vi "Autonomous Independent.vi"   [LabVIEW 2017]
doc: "This VI is called when autonomous begins, and will automatically be terminated when autonomous ends. You can carry out timed or sensor driven robot movement independently without needing to return to the caller."
uses:
  <vilib>/Rock Robotics/WPI/Utilities/WPI_GetSetVariantRefNum.vi
  <vilib>/Rock Robotics/Network Tables/NT Write Numeric Array.vi
  Robot Global Data.vi
  <vilib>/addons/control/pid/pid.llb/PID (DBL).vi
  <vilib>/addons/control/pid/NI_PID_pid.lvlib
panel:
  # "Be sure to right-click and choose Data Operations>>Make Current Value default if you want to save the array values with the VI"
types:
  T1 = typedef "WPI_JoystickDevRef.ctl" = cluster{"Device":T2}
  T2 = typedef "WPI_JoystickDeviceEnum.ctl" = enum16{"USB 0", "USB 1", "USB 2", "USB 3", "USB 4", "USB 5"}
  T3 = typedef "WPI_MotorControlDeviceRef.ctl" = cluster{"DeviceStatus":errorcluster, "Type":T4, "PWM":cluster{"PWM Channel":T5, "DeadBand":T6}, "CAN":cluster{"Device Number":u8, "SetOutput VI Ref":variant, "GetOutput VI Ref":variant, "Enable VI Ref":variant, "Disable VI Ref":variant, "Data":variant}, "Invert":bool, "DIO PWM":cluster{"PWM \"Enable\" Channel":T5, "DIOChannel":T7, "PWM Rate":dbl}}
  T4 = typedef "WPI_MotorControlType.ctl" = enum16{"PWM", "CAN", "DIO PWM"}
  T5 = typedef "FPGA_DIOPWMChannel.ctl" = enum8{"PWM 0", "PWM 1", "PWM 2", "PWM 3", "PWM 4", "PWM 5", "PWM 6", "PWM 7", "PWM 8", "PWM 9", "PWM MXP 0", "PWM MXP 1", "PWM MXP 2", "PWM MXP 3", "PWM MXP 4", "PWM MXP 5", "PWM MXP 6", "PWM MXP 7", "PWM MXP 8", "PWM MXP 9", "Invalid"}
  T6 = typedef "WPI_PWMDeadband.ctl" = cluster{"Name":string, "maxPositivePwm":i32, "minPositivePwm":i32, "centerPwm":i32, "maxNegativePwm":i32, "minNegativePwm":i32, "angularRange":u16}
  T7 = typedef "FPGA_DIOChannel.ctl" = enum8{"DIO 0", "DIO 1", "DIO 2", "DIO 3", "DIO 4", "DIO 5", "DIO 6", "DIO 7", "DIO 8", "DIO 9", "DIO MXP 0", "DIO MXP 1", "DIO MXP 2", "DIO MXP 3", "DIO MXP 4", "DIO MXP 5", "DIO MXP 6", "DIO MXP 7", "DIO MXP 8", "DIO MXP 9", "DIO MXP 10", "DIO MXP 11", "DIO MXP 12", "DIO MXP 13", "DIO MXP 14", "DIO MXP 15", "SPI Port CS1", "SPI Port CS2", "SPI Port CS3", "SPI Port MISO", "SPI Port MOSI", "Invalid"}
  T8 = cluster{"proportional gain (Kc)":dbl, "integral time (Ti, min)":dbl, "derivative time (Td, min)":dbl}
  T9 = typedef "CTRE_PigeonIMU_DeviceRef.ctl" = cluster{"DeviceStatus":errorcluster, "Device Number":u8, "Type":T10, "Device ID":u32, "Handle":u64, "UsageFrame":u32, "Library Path":path}
  T10 = typedef "CTRE_PigeonIMU_ConnectionType.ctl" = u32
  T11 = typedef "WPI_RobotDriveDevRef.ctl" = cluster{"DevStatus":errorcluster, "Motors[]":T3[], "Square Inputs":bool, "Max Output":dbl}
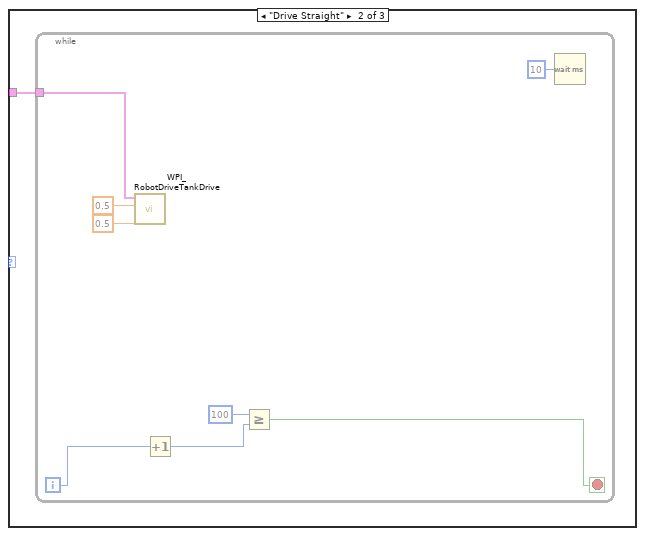
[diagram p2: hidden frame]
diagram:
  (unwired) "This function is run in parallel when the autonomous period begins. It will be terminated automatically when the period ends.\n\nNote that all Driver Station inputs are automatically latched and will not change once auto begins."
  # "This gives you the joystick value\nthat is often the throttle"
  # "Use time and/or sensors to control how the robot drives."
  n1 = call <vilib>:"WPI_JoystickRefNum Registry Get.vi"("refnum name"="Joystick 0") -> ("JoystickDevRef"=w21:T1)  [unwired: 1 in, 9 out]
  n2 = call <vilib>:"WPI_JoystickGetValues.vi"("JoystickDevRef"=w21) -> ("Buttons"=w19:bool[], "Axes"=w20:dbl[])  [unwired: 6 in, 3 out]
  n3 = call-poly <vilib>:"NT Write Value.vi"("Numeric Array"=w20, "Name"="Joystick 0/Axes") -> ()  [unwired: 9 in, 1 out]
  n4 = call <vilib>:"WPI_MotorControlRefNum Registry Get.vi"("refnum name"="LeftMaster") -> ("error out"=w14:errorcluster, "MotorControlDevRef"=w13:T3)  [unwired: 9 in]
  n5 = call <vilib>:"WPI_MotorControlRefNum Registry Get.vi"("refnum name"="RightMaster") -> ("error out"=w12:errorcluster, "MotorControlDevRef"=w11:T3)  [unwired: 9 in]
  n6 = Index Array(array=w19) -> (element #1=w9:bool, element #2=w5:bool, element #3=w2:bool)  [unwired: 8 in, 5 out]
  n7 = Select(t=enum16{"", "LEFT", "NONE", "RIGHT", "CENTER"}."CENTER", s=w2, f=enum16{"", "LEFT", "NONE", "RIGHT", "CENTER"}."NONE") -> (s? t:f=w4:enum16{"", "LEFT", "NONE", "RIGHT", "CENTER"})
  n8 = Select(t=enum16{"", "LEFT", "NONE", "RIGHT", "CENTER"}."RIGHT", s=w5, f=w4) -> (s? t:f=w7:enum16{"", "LEFT", "NONE", "RIGHT", "CENTER"})
  n9 = Select(t=enum16{"", "LEFT", "NONE", "RIGHT", "CENTER"}."LEFT", s=w9, f=w7) -> (s? t:f=w8:enum16{"", "LEFT", "NONE", "RIGHT", "CENTER"})
  n10 = case shown="\"LEFT\"" w8 {
    tunnel: w11 -> [_ w28 _ _]
    tunnel: w12 -> [_ w27 _ _]
    tunnel: w13 -> [_ w26 _ _]
    tunnel: w14 -> [_ w25 _ _]
    frame "NONE", Default {
    }
    frame "LEFT" {
      n11 = call <vilib>:"WPI_DriverStationGame Specific Data.vi"() -> ("Game Specific Data"=w24:string)  [unwired: 11 in]
      n12 = String Subset(string=w24, length (rest)=2 ("length (rest)")) -> (substring=w22:string)  [unwired: 1 in]
      n13 = case shown="\"LL\"" w22 {
        tunnel: w28 -> [_ w84 w323 _ _]
        tunnel: w27 -> [_ w70 w322 _ _]
        tunnel: w26 -> [_ w69 w321 _ _]
        tunnel: w25 -> [_ w68 w320 _ _]
        frame "None", Default {
        }
        frame "LL" {
          n14 = while {
            tunnel: [w230] -> w83
            tunnel: w84 -> [w230]
            tunnel: [w229] -> w67
            tunnel: w70 -> [w229]
            tunnel: [w228] -> w63
            tunnel: w69 -> [w228]
            tunnel: [w227] -> w62
            tunnel: w68 -> [w227]
            i -> [w236]
            stop <- w235 stop-if-true
            n15 = call "CTRE_PigeonIMU_RefNumRegistryGet.vi"("refnum name"="Pigeon") -> ("PigeonIMUDevRef"=w233:T9)  [unwired: 9 in, 1 out]
            n16 = Increment(x=w236) -> (x+1=w238:i32)
            n17 = call "CTRE_PigeonIMU_SetYaw.vi"("Value"=0.0, "PigeonIMUDevRef"=w233) -> ()  [unwired: 8 in, 2 out]
            n18 = Greater?(x=w238, y=1) -> (0:w235:bool)
            n19 = Wait (ms)(milliseconds to wait=u32 20) -> ()  [unwired: 1 out]
          }
          n20 = while {
            tunnel: [w272] -> w82
            tunnel: w83 -> [w272]
            tunnel: [w271] -> w66
            tunnel: w67 -> [w271]
            tunnel: [w270] -> w61
            tunnel: w63 -> [w270]
            tunnel: [w269] -> w60
            tunnel: w62 -> [w269]
            i -> [w275]
            stop <- w274 stop-if-true
            n21 = Wait (ms)(milliseconds to wait=u32 20) -> ()  [unwired: 1 out]
            n22 = Increment(x=w275) -> (x+1=w277:i32)
            n23 = call <vilib>:"WPI_RobotDriveRefNum Registry Get.vi"("refnum name"="RobotDrive") -> ("RobotDriveDevRef"=w279:T11)  [unwired: 9 in, 1 out]
            n24 = Greater?(x=w277, y=75) -> (0:w274:bool)
            n25 = call <vilib>:"WPI_RobotDriveTankDrive.vi"("Right axis value"=0.78, "Left axis value"=-0.75, "RobotDriveDevRef"=w279) -> ()  [unwired: 6 in, 3 out]
          }
          n26 = while {
            tunnel: [w258] -> w81
            tunnel: w82 -> [w258]
            tunnel: [w257] -> w65
            tunnel: w66 -> [w257]
            tunnel: [w256] -> w59
            tunnel: w61 -> [w256]
            tunnel: [w255] -> w58
            tunnel: w60 -> [w255]
            i -> [w264]
            stop <- w263 stop-if-true
            n27 = call "CTRE_PigeonIMU_RefNumRegistryGet.vi"("refnum name"="Pigeon") -> ("PigeonIMUDevRef"=w261:T9)  [unwired: 9 in, 1 out]
            n28 = Increment(x=w264) -> (x+1=w266:i32)
            n29 = call "CTRE_PigeonIMU_SetYaw.vi"("Value"=0.0, "PigeonIMUDevRef"=w261) -> ()  [unwired: 8 in, 2 out]
            n30 = Greater?(x=w266, y=2) -> (0:w263:bool)
            n31 = Wait (ms)(milliseconds to wait=u32 20) -> ()  [unwired: 1 out]
          }
          n32 = while {
            tunnel: [w242] -> w80
            tunnel: w81 -> [w242]
            tunnel: [w241] -> w64
            tunnel: w65 -> [w241]
            tunnel: [w240] -> w57
            tunnel: w59 -> [w240]
            tunnel: [w239] -> w56
            tunnel: w58 -> [w239]
            i -> [w245]
            stop <- w243 stop-if-true
            n33 = global read "Robot Global Data.vi" "YAW"() -> (w249:dbl)
            n34 = Increment(x=w245) -> (x+1=w247:i32)
            n35 = call-poly <vilib>:"PID.vi"("output range"=cluster{"output high":dbl, "output low":dbl} {"output high"=0.5, "output low"=-0.5}, "PID gains"=T8 {"proportional gain (Kc)"=0.04, "integral time (Ti, min)"=0.0, "derivative time (Td, min)"=0.0}, "process variable"=w249, "setpoint"=-90.0) -> ("output"=w253:dbl)  [unwired: 6 in, 1 out]
            n36 = Greater?(x=w247, y=120) -> (0:w243:bool)
            n37 = call <vilib>:"WPI_RobotDriveRefNum Registry Get.vi"("refnum name"="RobotDrive") -> ("RobotDriveDevRef"=w252:T11)  [unwired: 9 in, 1 out]
            n38 = Wait (ms)(milliseconds to wait=u32 20) -> ()  [unwired: 1 out]
            n39 = call <vilib>:"WPI_RobotDriveTankDrive.vi"("Right axis value"=w253, "Left axis value"=w253, "RobotDriveDevRef"=w252) -> ()  [unwired: 6 in, 3 out]
          }
          n40 = while {
            tunnel: [w114] -> w79
            tunnel: w80 -> [w114]
            tunnel: [w113] -> w55
            tunnel: w64 -> [w113]
            tunnel: [w112] -> w54
            tunnel: w57 -> [w112]
            tunnel: [w111] -> w53
            tunnel: w56 -> [w111]
            i -> [w117]
            stop <- w116 stop-if-true
            n41 = Wait (ms)(milliseconds to wait=u32 20) -> ()  [unwired: 1 out]
            n42 = Increment(x=w117) -> (x+1=w119:i32)
            n43 = call <vilib>:"WPI_RobotDriveRefNum Registry Get.vi"("refnum name"="RobotDrive") -> ("RobotDriveDevRef"=w123:T11)  [unwired: 9 in, 1 out]
            n44 = Greater?(x=w119, y=20) -> (0:w116:bool)
            n45 = call <vilib>:"WPI_RobotDriveTankDrive.vi"("Right axis value"=0.5, "Left axis value"=-0.5, "RobotDriveDevRef"=w123) -> ()  [unwired: 6 in, 3 out]
          }
          n46 = while {
            tunnel: [w88] -> w78
            tunnel: w79 -> [w88]
            tunnel: [w87] -> w52
            tunnel: w55 -> [w87]
            tunnel: [w86] -> w51
            tunnel: w54 -> [w86]
            tunnel: [w85] -> w50
            tunnel: w53 -> [w85]
            i -> [w91]
            stop <- w90 stop-if-true
            n47 = Wait (ms)(milliseconds to wait=u32 20) -> ()  [unwired: 1 out]
            n48 = Increment(x=w91) -> (x+1=w93:i32)
            n49 = call <vilib>:"WPI_RobotDriveRefNum Registry Get.vi"("refnum name"="RobotDrive") -> ("RobotDriveDevRef"=w97:T11)  [unwired: 9 in, 1 out]
            n50 = Greater?(x=w93, y=20) -> (0:w90:bool)
            n51 = call <vilib>:"WPI_RobotDriveTankDrive.vi"("Right axis value"=-0.5, "Left axis value"=0.5, "RobotDriveDevRef"=w97) -> ()  [unwired: 6 in, 3 out]
          }
          n52 = while {
            tunnel: [w214] -> w77
            tunnel: w78 -> [w214]
            tunnel: [w213] -> w49
            tunnel: w52 -> [w213]
            tunnel: [w212] -> w48
            tunnel: w51 -> [w212]
            tunnel: [w211] -> w47
            tunnel: w50 -> [w211]
            i -> [w217]
            stop <- w215 stop-if-true
            n53 = global read "Robot Global Data.vi" "YAW"() -> (w221:dbl)
            n54 = Increment(x=w217) -> (x+1=w219:i32)
            n55 = call-poly <vilib>:"PID.vi"("output range"=cluster{"output high":dbl, "output low":dbl} {"output high"=0.5, "output low"=-0.5}, "PID gains"=T8 {"proportional gain (Kc)"=0.04, "integral time (Ti, min)"=0.0, "derivative time (Td, min)"=0.0}, "process variable"=w221, "setpoint"=0.0) -> ("output"=w225:dbl)  [unwired: 6 in, 1 out]
            n56 = Greater?(x=w219, y=120) -> (0:w215:bool)
            n57 = call <vilib>:"WPI_RobotDriveRefNum Registry Get.vi"("refnum name"="RobotDrive") -> ("RobotDriveDevRef"=w224:T11)  [unwired: 9 in, 1 out]
            n58 = Wait (ms)(milliseconds to wait=u32 20) -> ()  [unwired: 1 out]
            n59 = call <vilib>:"WPI_RobotDriveTankDrive.vi"("Right axis value"=w225, "Left axis value"=w225, "RobotDriveDevRef"=w224) -> ()  [unwired: 6 in, 3 out]
          }
          n60 = while {
            tunnel: [w201] -> w76
            tunnel: w77 -> [w201]
            tunnel: [w200] -> w46
            tunnel: w49 -> [w200]
            tunnel: [w199] -> w45
            tunnel: w48 -> [w199]
            tunnel: [w198] -> w44
            tunnel: w47 -> [w198]
            i -> [w204]
            stop <- w203 stop-if-true
            n61 = Wait (ms)(milliseconds to wait=u32 20) -> ()  [unwired: 1 out]
            n62 = Increment(x=w204) -> (x+1=w206:i32)
            n63 = call <vilib>:"WPI_RobotDriveRefNum Registry Get.vi"("refnum name"="RobotDrive") -> ("RobotDriveDevRef"=w210:T11)  [unwired: 9 in, 1 out]
            n64 = Greater?(x=w206, y=40) -> (0:w203:bool)
            n65 = call <vilib>:"WPI_RobotDriveTankDrive.vi"("Right axis value"=0.8, "Left axis value"=-0.75, "RobotDriveDevRef"=w210) -> ()  [unwired: 6 in, 3 out]
          }
          n66 = while {
            tunnel: [w185] -> w75
            tunnel: w76 -> [w185]
            tunnel: [w184] -> w43
            tunnel: w46 -> [w184]
            tunnel: [w183] -> w42
            tunnel: w45 -> [w183]
            tunnel: [w182] -> w41
            tunnel: w44 -> [w182]
            i -> [w188]
            stop <- w186 stop-if-true
            n67 = global read "Robot Global Data.vi" "YAW"() -> (w192:dbl)
            n68 = Increment(x=w188) -> (x+1=w190:i32)
            n69 = call-poly <vilib>:"PID.vi"("output range"=cluster{"output high":dbl, "output low":dbl} {"output high"=0.5, "output low"=-0.5}, "PID gains"=T8 {"proportional gain (Kc)"=0.02, "integral time (Ti, min)"=0.0, "derivative time (Td, min)"=0.0}, "process variable"=w192, "setpoint"=-90.0) -> ("output"=w196:dbl)  [unwired: 6 in, 1 out]
            n70 = Greater?(x=w190, y=100) -> (0:w186:bool)
            n71 = call <vilib>:"WPI_RobotDriveRefNum Registry Get.vi"("refnum name"="RobotDrive") -> ("RobotDriveDevRef"=w195:T11)  [unwired: 9 in, 1 out]
            n72 = Wait (ms)(milliseconds to wait=u32 20) -> ()  [unwired: 1 out]
            n73 = call <vilib>:"WPI_RobotDriveTankDrive.vi"("Right axis value"=w196, "Left axis value"=w196, "RobotDriveDevRef"=w195) -> ()  [unwired: 6 in, 3 out]
          }
          n74 = while {
            tunnel: [w127] -> w74
            tunnel: w75 -> [w127]
            tunnel: [w126] -> w40
            tunnel: w43 -> [w126]
            tunnel: [w125] -> w39
            tunnel: w42 -> [w125]
            tunnel: [w124] -> w38
            tunnel: w41 -> [w124]
            i -> [w130]
            stop <- w129 stop-if-true
            n75 = Wait (ms)(milliseconds to wait=u32 20) -> ()  [unwired: 1 out]
            n76 = Increment(x=w130) -> (x+1=w132:i32)
            n77 = call <vilib>:"WPI_RobotDriveRefNum Registry Get.vi"("refnum name"="RobotDrive") -> ("RobotDriveDevRef"=w136:T11)  [unwired: 9 in, 1 out]
            n78 = Greater?(x=w132, y=30) -> (0:w129:bool)
            n79 = call <vilib>:"WPI_RobotDriveTankDrive.vi"("Right axis value"=0.5, "Left axis value"=-0.45, "RobotDriveDevRef"=w136) -> ()  [unwired: 6 in, 3 out]
          }
          n80 = while {
            tunnel: [w101] -> w73
            tunnel: w74 -> [w101]
            tunnel: [w100] -> w37
            tunnel: w40 -> [w100]
            tunnel: [w99] -> w36
            tunnel: w39 -> [w99]
            tunnel: [w98] -> w35
            tunnel: w38 -> [w98]
            i -> [w104]
            stop <- w103 stop-if-true
            n81 = Wait (ms)(milliseconds to wait=u32 20) -> ()  [unwired: 1 out]
            n82 = Increment(x=w104) -> (x+1=w106:i32)
            n83 = call <vilib>:"WPI_RobotDriveRefNum Registry Get.vi"("refnum name"="RobotDrive") -> ("RobotDriveDevRef"=w110:T11)  [unwired: 9 in, 1 out]
            n84 = Greater?(x=w106, y=20) -> (0:w103:bool)
            n85 = call <vilib>:"WPI_RobotDriveTankDrive.vi"("Right axis value"=-0.5, "Left axis value"=0.45, "RobotDriveDevRef"=w110) -> ()  [unwired: 6 in, 3 out]
          }
          n86 = while {
            tunnel: [w169] -> w72
            tunnel: w73 -> [w169]
            tunnel: [w168] -> w34
            tunnel: w37 -> [w168]
            tunnel: [w167] -> w33
            tunnel: w36 -> [w167]
            tunnel: [w166] -> w32
            tunnel: w35 -> [w166]
            i -> [w172]
            stop <- w170 stop-if-true
            n87 = global read "Robot Global Data.vi" "YAW"() -> (w176:dbl)
            n88 = Increment(x=w172) -> (x+1=w174:i32)
            n89 = call-poly <vilib>:"PID.vi"("output range"=cluster{"output high":dbl, "output low":dbl} {"output high"=0.5, "output low"=-0.5}, "PID gains"=T8 {"proportional gain (Kc)"=0.04, "integral time (Ti, min)"=0.0, "derivative time (Td, min)"=0.0}, "process variable"=w176, "setpoint"=10.0) -> ("output"=w180:dbl)  [unwired: 6 in, 1 out]
            n90 = Greater?(x=w174, y=120) -> (0:w170:bool)
            n91 = call <vilib>:"WPI_RobotDriveRefNum Registry Get.vi"("refnum name"="RobotDrive") -> ("RobotDriveDevRef"=w179:T11)  [unwired: 9 in, 1 out]
            n92 = Wait (ms)(milliseconds to wait=u32 20) -> ()  [unwired: 1 out]
            n93 = call <vilib>:"WPI_RobotDriveTankDrive.vi"("Right axis value"=w180, "Left axis value"=w180, "RobotDriveDevRef"=w179) -> ()  [unwired: 6 in, 3 out]
          }
          n94 = while {
            tunnel: [w156] -> w71
            tunnel: w72 -> [w156]
            tunnel: [w155] -> w31
            tunnel: w34 -> [w155]
            tunnel: [w154] -> w30
            tunnel: w33 -> [w154]
            tunnel: [w153] -> w29
            tunnel: w32 -> [w153]
            i -> [w159]
            stop <- w158 stop-if-true
            n95 = Wait (ms)(milliseconds to wait=u32 20) -> ()  [unwired: 1 out]
            n96 = Increment(x=w159) -> (x+1=w161:i32)
            n97 = call <vilib>:"WPI_RobotDriveRefNum Registry Get.vi"("refnum name"="RobotDrive") -> ("RobotDriveDevRef"=w165:T11)  [unwired: 9 in, 1 out]
            n98 = Greater?(x=w161, y=50) -> (0:w158:bool)
            n99 = call <vilib>:"WPI_RobotDriveTankDrive.vi"("Right axis value"=0.8, "Left axis value"=-0.75, "RobotDriveDevRef"=w165) -> ()  [unwired: 6 in, 3 out]
          }
          n100 = while {
            tunnel: [w140] -> _
            tunnel: w71 -> [w140]
            tunnel: [w139] -> _
            tunnel: w31 -> [w139]
            tunnel: [w138] -> _
            tunnel: w30 -> [w138]
            tunnel: [w137] -> _
            tunnel: w29 -> [w137]
            i -> [w143]
            stop <- w141 stop-if-true
            n101 = global read "Robot Global Data.vi" "YAW"() -> (w147:dbl)
            n102 = Increment(x=w143) -> (x+1=w145:i32)
            n103 = call-poly <vilib>:"PID.vi"("output range"=cluster{"output high":dbl, "output low":dbl} {"output high"=0.5, "output low"=-0.5}, "PID gains"=T8 {"proportional gain (Kc)"=0.02, "integral time (Ti, min)"=0.0, "derivative time (Td, min)"=0.0}, "process variable"=w147, "setpoint"=-80.0) -> ("output"=w151:dbl)  [unwired: 6 in, 1 out]
            n104 = Greater?(x=w145, y=120) -> (0:w141:bool)
            n105 = call <vilib>:"WPI_RobotDriveRefNum Registry Get.vi"("refnum name"="RobotDrive") -> ("RobotDriveDevRef"=w150:T11)  [unwired: 9 in, 1 out]
            n106 = Wait (ms)(milliseconds to wait=u32 20) -> ()  [unwired: 1 out]
            n107 = call <vilib>:"WPI_RobotDriveTankDrive.vi"("Right axis value"=w151, "Left axis value"=w151, "RobotDriveDevRef"=w150) -> ()  [unwired: 6 in, 3 out]
          }
        }
        frame "LR" {
          n108 = while {
            tunnel: [w535] -> w347
            tunnel: w323 -> [w535]
            tunnel: [w534] -> w341
            tunnel: w322 -> [w534]
            tunnel: [w533] -> w337
            tunnel: w321 -> [w533]
            tunnel: [w532] -> w336
            tunnel: w320 -> [w532]
            i -> [w541]
            stop <- w540 stop-if-true
            n109 = call "CTRE_PigeonIMU_RefNumRegistryGet.vi"("refnum name"="Pigeon") -> ("PigeonIMUDevRef"=w538:T9)  [unwired: 9 in, 1 out]
            n110 = Increment(x=w541) -> (x+1=w543:i32)
            n111 = call "CTRE_PigeonIMU_SetYaw.vi"("Value"=0.0, "PigeonIMUDevRef"=w538) -> ()  [unwired: 8 in, 2 out]
            n112 = Greater?(x=w543, y=1) -> (0:w540:bool)
            n113 = Wait (ms)(milliseconds to wait=u32 20) -> ()  [unwired: 1 out]
          }
          n114 = while {
            tunnel: [w575] -> w346
            tunnel: w347 -> [w575]
            tunnel: [w574] -> w340
            tunnel: w341 -> [w574]
            tunnel: [w573] -> w335
            tunnel: w337 -> [w573]
            tunnel: [w572] -> w334
            tunnel: w336 -> [w572]
            i -> [w578]
            stop <- w577 stop-if-true
            n115 = Wait (ms)(milliseconds to wait=u32 20) -> ()  [unwired: 1 out]
            n116 = Increment(x=w578) -> (x+1=w580:i32)
            n117 = call <vilib>:"WPI_RobotDriveRefNum Registry Get.vi"("refnum name"="RobotDrive") -> ("RobotDriveDevRef"=w584:T11)  [unwired: 9 in, 1 out]
            n118 = Greater?(x=w580, y=130) -> (0:w577:bool)
            n119 = call <vilib>:"WPI_RobotDriveTankDrive.vi"("Right axis value"=0.78, "Left axis value"=-0.75, "RobotDriveDevRef"=w584) -> ()  [unwired: 6 in, 3 out]
          }
          n120 = while {
            tunnel: [w563] -> w345
            tunnel: w346 -> [w563]
            tunnel: [w562] -> w339
            tunnel: w340 -> [w562]
            tunnel: [w561] -> w333
            tunnel: w335 -> [w561]
            tunnel: [w560] -> w332
            tunnel: w334 -> [w560]
            i -> [w569]
            stop <- w568 stop-if-true
            n121 = call "CTRE_PigeonIMU_RefNumRegistryGet.vi"("refnum name"="Pigeon") -> ("PigeonIMUDevRef"=w566:T9)  [unwired: 9 in, 1 out]
            n122 = Increment(x=w569) -> (x+1=w571:i32)
            n123 = call "CTRE_PigeonIMU_SetYaw.vi"("Value"=0.0, "PigeonIMUDevRef"=w566) -> ()  [unwired: 8 in, 2 out]
            n124 = Greater?(x=w571, y=2) -> (0:w568:bool)
            n125 = Wait (ms)(milliseconds to wait=u32 20) -> ()  [unwired: 1 out]
          }
          n126 = while {
            tunnel: [w547] -> w344
            tunnel: w345 -> [w547]
            tunnel: [w546] -> w338
            tunnel: w339 -> [w546]
            tunnel: [w545] -> w331
            tunnel: w333 -> [w545]
            tunnel: [w544] -> w330
            tunnel: w332 -> [w544]
            i -> [w550]
            stop <- w548 stop-if-true
            n127 = global read "Robot Global Data.vi" "YAW"() -> (w554:dbl)
            n128 = Increment(x=w550) -> (x+1=w552:i32)
            n129 = call-poly <vilib>:"PID.vi"("output range"=cluster{"output high":dbl, "output low":dbl} {"output high"=0.5, "output low"=-0.5}, "PID gains"=T8 {"proportional gain (Kc)"=0.04, "integral time (Ti, min)"=0.0, "derivative time (Td, min)"=0.0}, "process variable"=w554, "setpoint"=-90.0) -> ("output"=w558:dbl)  [unwired: 6 in, 1 out]
            n130 = Greater?(x=w552, y=140) -> (0:w548:bool)
            n131 = call <vilib>:"WPI_RobotDriveRefNum Registry Get.vi"("refnum name"="RobotDrive") -> ("RobotDriveDevRef"=w557:T11)  [unwired: 9 in, 1 out]
            n132 = Wait (ms)(milliseconds to wait=u32 20) -> ()  [unwired: 1 out]
            n133 = call <vilib>:"WPI_RobotDriveTankDrive.vi"("Right axis value"=w558, "Left axis value"=w558, "RobotDriveDevRef"=w557) -> ()  [unwired: 6 in, 3 out]
          }
          n134 = while {
            tunnel: [w506] -> w343
            tunnel: w344 -> [w506]
            tunnel: [w505] -> w329
            tunnel: w338 -> [w505]
            tunnel: [w504] -> w328
            tunnel: w331 -> [w504]
            tunnel: [w503] -> w327
            tunnel: w330 -> [w503]
            i -> [w509]
            stop <- w508 stop-if-true
            n135 = Wait (ms)(milliseconds to wait=u32 20) -> ()  [unwired: 1 out]
            n136 = Increment(x=w509) -> (x+1=w511:i32)
            n137 = call <vilib>:"WPI_RobotDriveRefNum Registry Get.vi"("refnum name"="RobotDrive") -> ("RobotDriveDevRef"=w515:T11)  [unwired: 9 in, 1 out]
            n138 = Greater?(x=w511, y=50) -> (0:w508:bool)
            n139 = call <vilib>:"WPI_RobotDriveTankDrive.vi"("Right axis value"=0.5, "Left axis value"=-0.45, "RobotDriveDevRef"=w515) -> ()  [unwired: 6 in, 3 out]
          }
          n140 = while {
            tunnel: [w493] -> w342
            tunnel: w343 -> [w493]
            tunnel: [w492] -> w326
            tunnel: w329 -> [w492]
            tunnel: [w491] -> w325
            tunnel: w328 -> [w491]
            tunnel: [w490] -> w324
            tunnel: w327 -> [w490]
            i -> [w496]
            stop <- w495 stop-if-true
            n141 = Wait (ms)(milliseconds to wait=u32 20) -> ()  [unwired: 1 out]
            n142 = Increment(x=w496) -> (x+1=w498:i32)
            n143 = call <vilib>:"WPI_RobotDriveRefNum Registry Get.vi"("refnum name"="RobotDrive") -> ("RobotDriveDevRef"=w502:T11)  [unwired: 9 in, 1 out]
            n144 = Greater?(x=w498, y=30) -> (0:w495:bool)
            n145 = call <vilib>:"WPI_RobotDriveTankDrive.vi"("Right axis value"=-0.5, "Left axis value"=0.45, "RobotDriveDevRef"=w502) -> ()  [unwired: 6 in, 3 out]
          }
          n146 = while {
            tunnel: [w519] -> w287
            tunnel: w342 -> [w519]
            tunnel: [w518] -> w286
            tunnel: w326 -> [w518]
            tunnel: [w517] -> w285
            tunnel: w325 -> [w517]
            tunnel: [w516] -> w284
            tunnel: w324 -> [w516]
            i -> [w522]
            stop <- w520 stop-if-true
            n147 = global read "Robot Global Data.vi" "YAW"() -> (w526:dbl)
            n148 = Increment(x=w522) -> (x+1=w524:i32)
            n149 = call-poly <vilib>:"PID.vi"("output range"=cluster{"output high":dbl, "output low":dbl} {"output high"=0.5, "output low"=-0.5}, "PID gains"=T8 {"proportional gain (Kc)"=0.03, "integral time (Ti, min)"=0.0, "derivative time (Td, min)"=0.0}, "process variable"=w526, "setpoint"=0.0) -> ("output"=w530:dbl)  [unwired: 6 in, 1 out]
            n150 = Greater?(x=w524, y=160) -> (0:w520:bool)
            n151 = call <vilib>:"WPI_RobotDriveRefNum Registry Get.vi"("refnum name"="RobotDrive") -> ("RobotDriveDevRef"=w529:T11)  [unwired: 9 in, 1 out]
            n152 = Wait (ms)(milliseconds to wait=u32 20) -> ()  [unwired: 1 out]
            n153 = call <vilib>:"WPI_RobotDriveTankDrive.vi"("Right axis value"=w530, "Left axis value"=w530, "RobotDriveDevRef"=w529) -> ()  [unwired: 6 in, 3 out]
          }
          n154 = while {
            tunnel: [w480] -> w319
            tunnel: w287 -> [w480]
            tunnel: [w479] -> w315
            tunnel: w286 -> [w479]
            tunnel: [w478] -> w314
            tunnel: w285 -> [w478]
            tunnel: [w477] -> w313
            tunnel: w284 -> [w477]
            i -> [w483]
            stop <- w482 stop-if-true
            n155 = Wait (ms)(milliseconds to wait=u32 20) -> ()  [unwired: 1 out]
            n156 = Increment(x=w483) -> (x+1=w485:i32)
            n157 = call <vilib>:"WPI_RobotDriveRefNum Registry Get.vi"("refnum name"="RobotDrive") -> ("RobotDriveDevRef"=w489:T11)  [unwired: 9 in, 1 out]
            n158 = Greater?(x=w485, y=100) -> (0:w482:bool)
            n159 = call <vilib>:"WPI_RobotDriveTankDrive.vi"("Right axis value"=0.6, "Left axis value"=-0.55, "RobotDriveDevRef"=w489) -> ()  [unwired: 6 in, 3 out]
          }
          n160 = while {
            tunnel: [w464] -> w318
            tunnel: w319 -> [w464]
            tunnel: [w463] -> w312
            tunnel: w315 -> [w463]
            tunnel: [w462] -> w311
            tunnel: w314 -> [w462]
            tunnel: [w461] -> w310
            tunnel: w313 -> [w461]
            i -> [w467]
            stop <- w465 stop-if-true
            n161 = global read "Robot Global Data.vi" "YAW"() -> (w471:dbl)
            n162 = Increment(x=w467) -> (x+1=w469:i32)
            n163 = call-poly <vilib>:"PID.vi"("output range"=cluster{"output high":dbl, "output low":dbl} {"output high"=0.5, "output low"=-0.5}, "PID gains"=T8 {"proportional gain (Kc)"=0.03, "integral time (Ti, min)"=0.0, "derivative time (Td, min)"=0.0}, "process variable"=w471, "setpoint"=-90.0) -> ("output"=w475:dbl)  [unwired: 6 in, 1 out]
            n164 = Greater?(x=w469, y=160) -> (0:w465:bool)
            n165 = call <vilib>:"WPI_RobotDriveRefNum Registry Get.vi"("refnum name"="RobotDrive") -> ("RobotDriveDevRef"=w474:T11)  [unwired: 9 in, 1 out]
            n166 = Wait (ms)(milliseconds to wait=u32 20) -> ()  [unwired: 1 out]
            n167 = call <vilib>:"WPI_RobotDriveTankDrive.vi"("Right axis value"=w475, "Left axis value"=w475, "RobotDriveDevRef"=w474) -> ()  [unwired: 6 in, 3 out]
          }
          n168 = while {
            tunnel: [w435] -> w317
            tunnel: w318 -> [w435]
            tunnel: [w434] -> w309
            tunnel: w312 -> [w434]
            tunnel: [w433] -> w308
            tunnel: w311 -> [w433]
            tunnel: [w432] -> w307
            tunnel: w310 -> [w432]
            i -> [w438]
            stop <- w437 stop-if-true
            n169 = Wait (ms)(milliseconds to wait=u32 20) -> ()  [unwired: 1 out]
            n170 = Increment(x=w438) -> (x+1=w440:i32)
            n171 = call <vilib>:"WPI_RobotDriveRefNum Registry Get.vi"("refnum name"="RobotDrive") -> ("RobotDriveDevRef"=w444:T11)  [unwired: 9 in, 1 out]
            n172 = Greater?(x=w440, y=50) -> (0:w437:bool)
            n173 = call <vilib>:"WPI_RobotDriveTankDrive.vi"("Right axis value"=0.5, "Left axis value"=-0.45, "RobotDriveDevRef"=w444) -> ()  [unwired: 6 in, 3 out]
          }
          n174 = while {
            tunnel: [w422] -> w316
            tunnel: w317 -> [w422]
            tunnel: [w421] -> w306
            tunnel: w309 -> [w421]
            tunnel: [w420] -> w305
            tunnel: w308 -> [w420]
            tunnel: [w419] -> w304
            tunnel: w307 -> [w419]
            i -> [w425]
            stop <- w424 stop-if-true
            n175 = Wait (ms)(milliseconds to wait=u32 20) -> ()  [unwired: 1 out]
            n176 = Increment(x=w425) -> (x+1=w427:i32)
            n177 = call <vilib>:"WPI_RobotDriveRefNum Registry Get.vi"("refnum name"="RobotDrive") -> ("RobotDriveDevRef"=w431:T11)  [unwired: 9 in, 1 out]
            n178 = Greater?(x=w427, y=30) -> (0:w424:bool)
            n179 = call <vilib>:"WPI_RobotDriveTankDrive.vi"("Right axis value"=-0.5, "Left axis value"=0.45, "RobotDriveDevRef"=w431) -> ()  [unwired: 6 in, 3 out]
          }
          n180 = while {
            tunnel: [w448] -> w303
            tunnel: w316 -> [w448]
            tunnel: [w447] -> w302
            tunnel: w306 -> [w447]
            tunnel: [w446] -> w301
            tunnel: w305 -> [w446]
            tunnel: [w445] -> w300
            tunnel: w304 -> [w445]
            i -> [w451]
            stop <- w449 stop-if-true
            n181 = global read "Robot Global Data.vi" "YAW"() -> (w455:dbl)
            n182 = Increment(x=w451) -> (x+1=w453:i32)
            n183 = call-poly <vilib>:"PID.vi"("output range"=cluster{"output high":dbl, "output low":dbl} {"output high"=0.5, "output low"=-0.5}, "PID gains"=T8 {"proportional gain (Kc)"=0.04, "integral time (Ti, min)"=0.0, "derivative time (Td, min)"=0.0}, "process variable"=w455, "setpoint"=-180.0) -> ("output"=w459:dbl)  [unwired: 6 in, 1 out]
            n184 = Greater?(x=w453, y=120) -> (0:w449:bool)
            n185 = call <vilib>:"WPI_RobotDriveRefNum Registry Get.vi"("refnum name"="RobotDrive") -> ("RobotDriveDevRef"=w458:T11)  [unwired: 9 in, 1 out]
            n186 = Wait (ms)(milliseconds to wait=u32 20) -> ()  [unwired: 1 out]
            n187 = call <vilib>:"WPI_RobotDriveTankDrive.vi"("Right axis value"=w459, "Left axis value"=w459, "RobotDriveDevRef"=w458) -> ()  [unwired: 6 in, 3 out]
          }
          n188 = while {
            tunnel: [w409] -> w299
            tunnel: w303 -> [w409]
            tunnel: [w408] -> w298
            tunnel: w302 -> [w408]
            tunnel: [w407] -> w297
            tunnel: w301 -> [w407]
            tunnel: [w406] -> w296
            tunnel: w300 -> [w406]
            i -> [w412]
            stop <- w411 stop-if-true
            n189 = Wait (ms)(milliseconds to wait=u32 20) -> ()  [unwired: 1 out]
            n190 = Increment(x=w412) -> (x+1=w414:i32)
            n191 = call <vilib>:"WPI_RobotDriveRefNum Registry Get.vi"("refnum name"="RobotDrive") -> ("RobotDriveDevRef"=w418:T11)  [unwired: 9 in, 1 out]
            n192 = Greater?(x=w414, y=60) -> (0:w411:bool)
            n193 = call <vilib>:"WPI_RobotDriveTankDrive.vi"("Right axis value"=0.6, "Left axis value"=-0.5, "RobotDriveDevRef"=w418) -> ()  [unwired: 6 in, 3 out]
          }
          n194 = while {
            tunnel: [w393] -> w291
            tunnel: w299 -> [w393]
            tunnel: [w392] -> w290
            tunnel: w298 -> [w392]
            tunnel: [w391] -> w289
            tunnel: w297 -> [w391]
            tunnel: [w390] -> w288
            tunnel: w296 -> [w390]
            i -> [w396]
            stop <- w394 stop-if-true
            n195 = global read "Robot Global Data.vi" "YAW"() -> (w400:dbl)
            n196 = Increment(x=w396) -> (x+1=w398:i32)
            n197 = call-poly <vilib>:"PID.vi"("output range"=cluster{"output high":dbl, "output low":dbl} {"output high"=0.5, "output low"=-0.5}, "PID gains"=T8 {"proportional gain (Kc)"=0.03, "integral time (Ti, min)"=0.0, "derivative time (Td, min)"=0.0}, "process variable"=w400, "setpoint"=-90.0) -> ("output"=w404:dbl)  [unwired: 6 in, 1 out]
            n198 = Greater?(x=w398, y=160) -> (0:w394:bool)
            n199 = call <vilib>:"WPI_RobotDriveRefNum Registry Get.vi"("refnum name"="RobotDrive") -> ("RobotDriveDevRef"=w403:T11)  [unwired: 9 in, 1 out]
            n200 = Wait (ms)(milliseconds to wait=u32 20) -> ()  [unwired: 1 out]
            n201 = call <vilib>:"WPI_RobotDriveTankDrive.vi"("Right axis value"=w404, "Left axis value"=w404, "RobotDriveDevRef"=w403) -> ()  [unwired: 6 in, 3 out]
          }
          n202 = while {
            tunnel: [w380] -> w295
            tunnel: w291 -> [w380]
            tunnel: [w379] -> w294
            tunnel: w290 -> [w379]
            tunnel: [w378] -> w293
            tunnel: w289 -> [w378]
            tunnel: [w377] -> w292
            tunnel: w288 -> [w377]
            i -> [w383]
            stop <- w382 stop-if-true
            n203 = Wait (ms)(milliseconds to wait=u32 20) -> ()  [unwired: 1 out]
            n204 = Increment(x=w383) -> (x+1=w385:i32)
            n205 = call <vilib>:"WPI_RobotDriveRefNum Registry Get.vi"("refnum name"="RobotDrive") -> ("RobotDriveDevRef"=w389:T11)  [unwired: 9 in, 1 out]
            n206 = Greater?(x=w385, y=50) -> (0:w382:bool)
            n207 = call <vilib>:"WPI_RobotDriveTankDrive.vi"("Right axis value"=0.5, "Left axis value"=-0.5, "RobotDriveDevRef"=w389) -> ()  [unwired: 6 in, 3 out]
          }
          n208 = while {
            tunnel: [w367] -> w283
            tunnel: w295 -> [w367]
            tunnel: [w366] -> w282
            tunnel: w294 -> [w366]
            tunnel: [w365] -> w281
            tunnel: w293 -> [w365]
            tunnel: [w364] -> w280
            tunnel: w292 -> [w364]
            i -> [w370]
            stop <- w369 stop-if-true
            n209 = Wait (ms)(milliseconds to wait=u32 20) -> ()  [unwired: 1 out]
            n210 = Increment(x=w370) -> (x+1=w372:i32)
            n211 = call <vilib>:"WPI_RobotDriveRefNum Registry Get.vi"("refnum name"="RobotDrive") -> ("RobotDriveDevRef"=w376:T11)  [unwired: 9 in, 1 out]
            n212 = Greater?(x=w372, y=30) -> (0:w369:bool)
            n213 = call <vilib>:"WPI_RobotDriveTankDrive.vi"("Right axis value"=-0.5, "Left axis value"=0.45, "RobotDriveDevRef"=w376) -> ()  [unwired: 6 in, 3 out]
          }
          n214 = while {
            tunnel: [w351] -> _
            tunnel: w283 -> [w351]
            tunnel: [w350] -> _
            tunnel: w282 -> [w350]
            tunnel: [w349] -> _
            tunnel: w281 -> [w349]
            tunnel: [w348] -> _
            tunnel: w280 -> [w348]
            i -> [w354]
            stop <- w352 stop-if-true
            n215 = global read "Robot Global Data.vi" "YAW"() -> (w358:dbl)
            n216 = Increment(x=w354) -> (x+1=w356:i32)
            n217 = call-poly <vilib>:"PID.vi"("output range"=cluster{"output high":dbl, "output low":dbl} {"output high"=0.5, "output low"=-0.5}, "PID gains"=T8 {"proportional gain (Kc)"=0.03, "integral time (Ti, min)"=0.0, "derivative time (Td, min)"=0.0}, "process variable"=w358, "setpoint"=0.0) -> ("output"=w362:dbl)  [unwired: 6 in, 1 out]
            n218 = Greater?(x=w356, y=100) -> (0:w352:bool)
            n219 = call <vilib>:"WPI_RobotDriveRefNum Registry Get.vi"("refnum name"="RobotDrive") -> ("RobotDriveDevRef"=w361:T11)  [unwired: 9 in, 1 out]
            n220 = Wait (ms)(milliseconds to wait=u32 20) -> ()  [unwired: 1 out]
            n221 = call <vilib>:"WPI_RobotDriveTankDrive.vi"("Right axis value"=w362, "Left axis value"=w362, "RobotDriveDevRef"=w361) -> ()  [unwired: 6 in, 3 out]
          }
        }
        frame "RR" {
        }
        frame "RL" {
        }
      }
    }
    frame "RIGHT" {
    }
    frame "CENTER" {
    }
  }
  n222 = disable-structure shown="Disabled" {
    disable-tunnel: _ -> [w589 _]
    frame Disabled {
      (unwired) enum16{"Turn", "Drive Straight", "Nothing"}."Nothing"
      (unwired) enum16{"Turn", "Drive Straight", "Nothing"}."Turn"
      (unwired) enum16{"Drive Straight", "None", "Turn 90"}."Drive Straight"
      n223 = call <vilib>:"WPI_JoystickGetValues.vi"("JoystickDevRef"=w589) -> ("Buttons"=w588:bool[])  [unwired: 6 in, 4 out]
      n224 = Index Array(array=w588, index #1=1 ("index"), index #2=2 ("index")) -> ()  [unwired: 2 out]
      n225 = call <vilib>:"WPI_RobotDriveRefNum Registry Get.vi"("refnum name"="RobotDrive") -> ("RobotDriveDevRef"=w590:T11)  [unwired: 9 in, 1 out]
      n226 = case shown="\"Turn\", Default" enum16{"Turn", "Drive Straight", "Nothing"}."Drive Straight" {
        tunnel: w590 -> [_ w592 _]
        frame "Turn", Default {
        }
        frame "Drive Straight" {
          n227 = while {
            tunnel: w592 -> [w593]
            i -> [w600]
            stop <- w597 stop-if-true
            n228 = call <vilib>:"WPI_RobotDriveTankDrive.vi"("Right axis value"=0.5, "Left axis value"=0.5, "RobotDriveDevRef"=w593) -> ()  [unwired: 6 in, 3 out]
            n229 = Increment(x=w600) -> (x+1=w599:i32)
            n230 = Greater Or Equal?(x=100, y=w599) -> (x >= y?=w597:bool)
            n231 = Wait (ms)(milliseconds to wait=u32 10) -> ()  [unwired: 1 out]
          }
        }
        frame "Nothing" {
        }
      }
    }
    frame Enabled {
    }
  }
